vi "FPGA Main.vi"   [LabVIEW 2018]
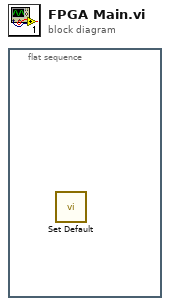
[diagram p0: block diagram]
diagram:
  n1 = flat-sequence {
    frame #0 {
      n2 = call "Set Default.vi"() -> ()  [unwired: 6 in]
    }
  }
